vi "dropdownlist global.vi"() -> ()   [LabVIEW 2014]
panel:
  in  "Ring":u16(ring)
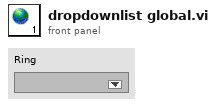
[diagram p1: front panel]
diagram:
